vi "cRIO debug.vi"() -> ()   [LabVIEW 2009]
uses:
  UDP Lib/UDP Network Location.ctl
panel:
  out "B":bool
  out "Network Location":T1
  out "Waveform Graph":u16[](graph)
  in  "stop":bool
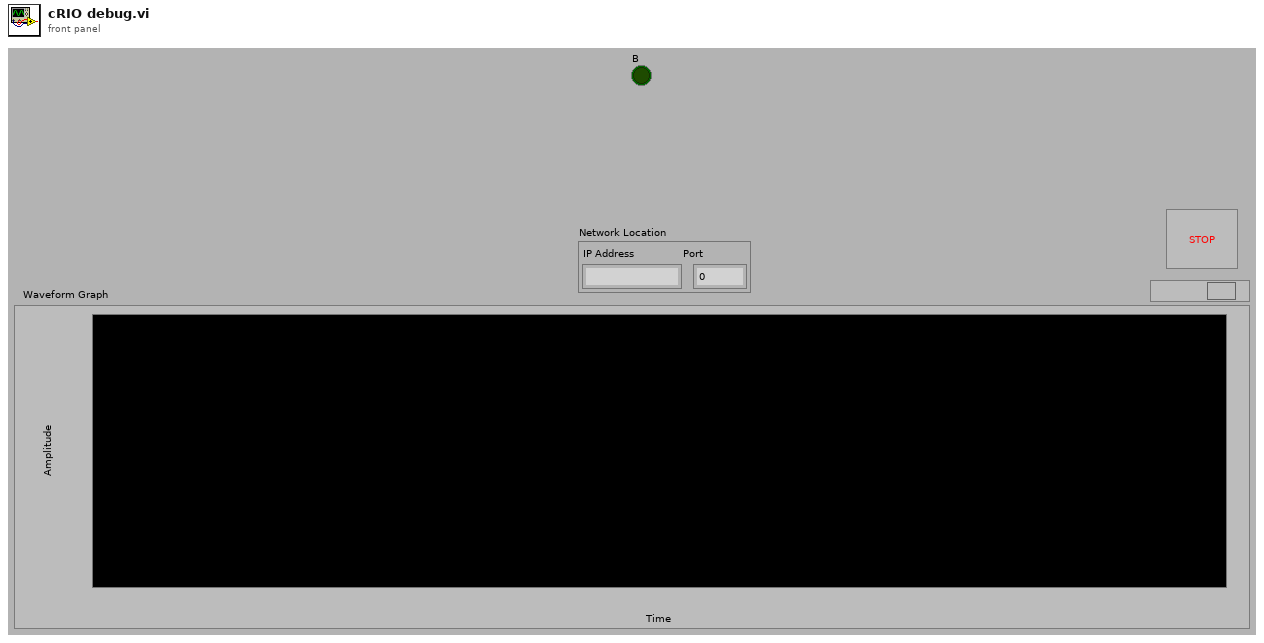
[diagram p1: front panel]
types:
  T1 = typedef "UDP Network Location.ctl" = cluster{"IP Address":string, "Port":u16}
  T2 = typedef "UDP Base.ctl" = cluster{"UDP Session":refnum<k16>, "UDP Socket Params":T3}
  T3 = typedef "UDP Socket Params.ctl" = cluster{"Local Port":u16, "Read Timeout":i32, "Write Timeout":i32}
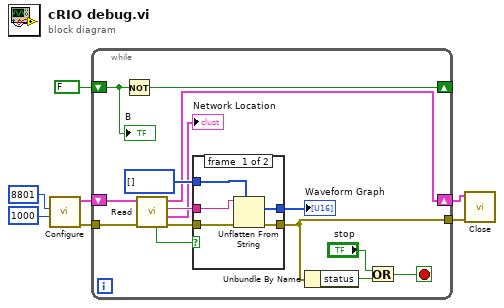
[diagram p0: block diagram]
diagram:
  n1 = call "Configure.vi"("Read Timeout"=1000, "Local Port"=u16 8801) -> ("error out"=w6:errorcluster, "UDP Base out"=w7:T2)  [unwired: 8 in]
  n2 = while {
    tunnel: w6 -> [w15]
    tunnel: [w18] -> w4
    shift-right: [w12] -> w3
    shift-left: w7 -> [w16]
    shift-right: [w8] -> _
    shift-left: FALSE ("Timeout") -> [w9]
    stop <- w19 stop-if-true
    n3 = Not(x=w9) -> (.not. x?=w8:bool)
    n4 = call "Read.vi"("error in (no error)"=w15, "UDP Base in"=w16) -> ("error out"=w14:errorcluster, "Network Location"=→"Network Location":T1, "Receive Data"=w13:string, "UDP Base out"=w12:T2, "Timeout"=w11:bool)  [unwired: 4 in, 1 out]
    n5 = case shown="True" w11 {
      tunnel: u16[] [] -> [w27 w29]
      tunnel: [w26 w29] -> w20
      tunnel: [w25 w28] -> w18
      tunnel: w14 -> [w24 w28]
      tunnel: w13 -> [w23 _]
      frame #0 {
        n6 = Unflatten From String(type=w27, binary string=w23, error in (no error)=w24) -> (value=w26:u16[], error out=w25:errorcluster)  [unwired: 2 in, 1 out]
      }
      frame #1 {
      }
    }
    "Waveform Graph" <- w20
    n7 = Unbundle By Name(w18) -> ("status"=w17:bool)
    n8 = Or(x="stop", y=w17) -> (x .or. y?=w19:bool)
    "B" <- w9
  }
  n9 = call "Close.vi"("error in (no error)"=w4, "Cluster of class private data"=w3) -> ()  [unwired: 9 in, 1 out]
